vi "MathCad_Easy_Matrix_Get_2D.vi"(8 "error in (no error)":errorcluster, 9 "Variable  Name":string, 11 "Mathcad Reference":T1) -> (0 "error out":errorcluster, 1 "Array":dbl[][](array[numeric]) format="%.2f", 3 "Mathcad Reference":T1)   [LabVIEW 2015]
doc: "Gets the 2-D Matrix value in Mathcad. It gets the last definition of the variable.\n\nInputs\n Wrksht Ref--ActiveX Reference to Mathcad Worksheet Class\n Variable Name (String)--Name of Variable to get.\n\nOutputs\n Wrksht Ref--ActiveX Reference to Mathcad Worksheet Class \n Value (2-D Array of Doubles)--Value definition of the Variable in the Mathcad Worksheet."
uses:
  Mathcad Reference.ctl
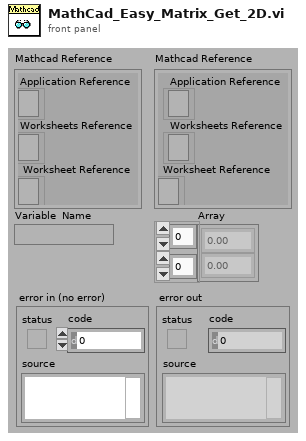
[diagram p1: front panel]
types:
  T1 = typedef "Mathcad Reference.ctl" = cluster{"Application Reference":refnum<k7>, "Worksheets Reference":refnum<k7>, " Worksheet Reference":refnum<k7>}
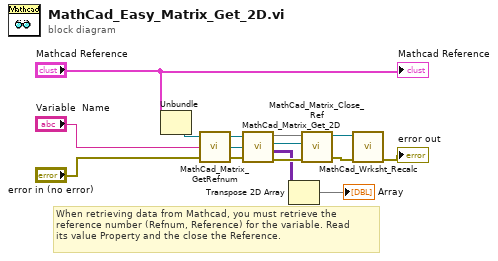
[diagram p0: block diagram]
diagram:
  # "When retrieving data from Mathcad, you must retrieve the \nreference number (Refnum, Reference) for the variable. Read \nits value Property and the close the Reference."
  n1 = Unbundle("Mathcad Reference") -> ("Worksheet Reference"=w2:refnum<k7>)  [unwired: 2 out]
  n2 = call "MathCad_Matrix_GetRefnum.vi"("error in (no error)"="error in (no error)", "Variable  Name"="Variable  Name", "Worksheet Reference In"=w2) -> ("error out"=w11:errorcluster, "Mathcad.IMatrixValue Refnum"=w12:refnum<k7>, "Worksheet Reference Out"=w13:refnum<k7>)
  n3 = call "MathCad_Matrix_Get_2D.vi"(0:w13, "Mathcad.IMatrixValue Refnum"=w12, "error out 2"=w11) -> (3:w10, "Mathcad.IMatrixValue Refnum"=w9:refnum<k7>, "Array"=w4:variant[][], "error out"=w8:errorcluster)
  n4 = Transpose 2D Array(2D array=w4) -> (transposed array=→"Array":variant[][])
  n5 = call "MathCad_Matrix_Close_Ref.vi"("error in"=w8, "Mathcad.IMatrixValue Reference"=w9, "IMathcadWorksheet Reference"=w10) -> ("error out"=w7:errorcluster, "IMathcadWorksheet Reference"=w6:refnum<k7>)  [unwired: 2 in]
  n6 = call "MathCad_Wrksht_Recalc.vi"("error in (no error)"=w7, "Worksheet Reference"=w6) -> ("error out"=→"error out":errorcluster)  [unwired: 8 in, 1 out]
  "Mathcad Reference" <- "Mathcad Reference"
